vi "Mars3D_autosort.vi"() -> ()   [LabVIEW 2013]
panel:
  in  "Autosize Parameter Set":T1(array[cluster])=[{"Autosize Parameter Set 2"=[{"Trigger Ch"=0, "Min Vel"=0.0, "MaxVel"=0.0, "Width"=0, "Pre Impuls"=0, "Post Impuls"=0, "Pitch"=0.0, "Name"="No Datafile selected", "Other Trigger"=FALSE, "Cross Corr"=FALSE, "Default"={"Freq"=0.0, "Vel"=0.0, "Acc"=0.0, "Stimulus"=""}}]}]
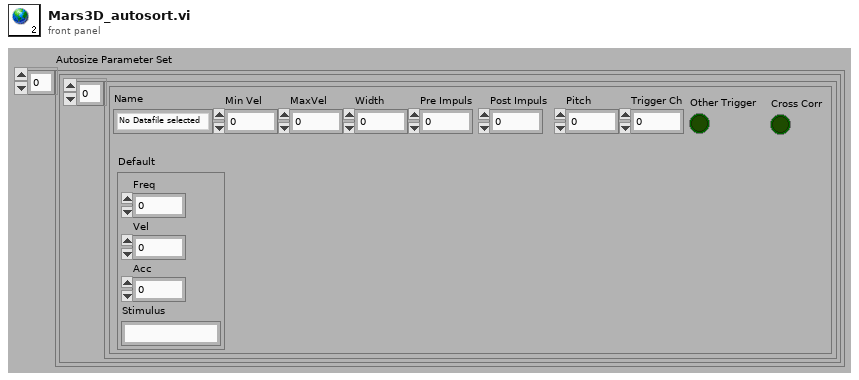
[diagram p1: front panel]
types:
  T1 = cluster{"Autosize Parameter Set 2":cluster{"Trigger Ch":i32, "Min Vel":dbl, "MaxVel":dbl, "Width":i32, "Pre Impuls":i32, "Post Impuls":i32, "Pitch":dbl, "Name":string, "Other Trigger":bool, "Cross Corr":bool, "Default":cluster{"Freq":dbl, "Vel":dbl, "Acc":dbl, "Stimulus":string}}[]}[]
diagram:
